vi "IR121206 Traitement Enr Npectre_SD.vi"(1 "Moyenne par pas":i8=4, 3 "resultat_input":dbl[](array[numeric])=array[24576 elements]) -> (0 "BgSig":dbl[][](array[numeric]), 2 "Ref-Bg":dbl[][](array[numeric]), 4 "BgRef":dbl[][](array[numeric]), 5 "Sig-Bg":dbl[][](array[numeric]))   [LabVIEW 2015]
panel:
  out "Graphe":dbl[](graph)
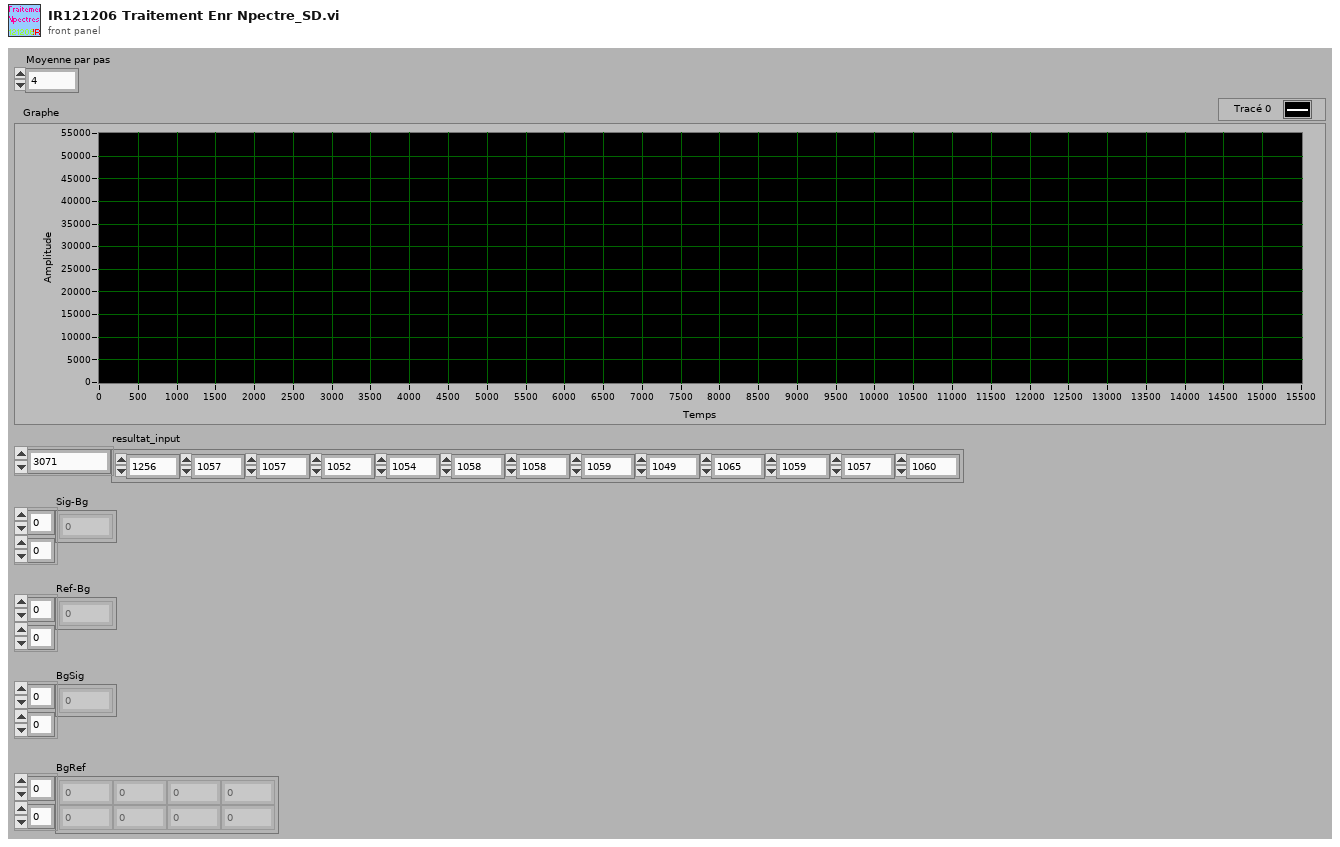
[diagram p1: front panel]
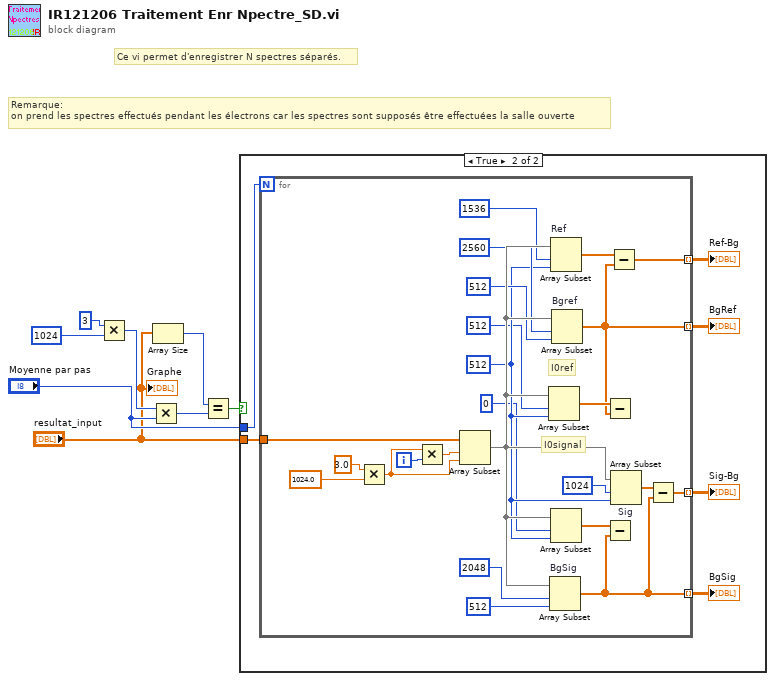
[diagram p0: block diagram]
diagram:
  # "Ce vi permet d'enregistrer N spectres séparés."
  # "Remarque: \non prend les spectres effectués pendant les électrons car les spectres sont supposés être effectuées la salle ouverte"
  n1 = Multiply(x=3, y=1024) -> (x*y=w6:i32)
  n2 = Multiply(x=w6, y="Moyenne par pas") -> (x*y=w4:i32)
  n3 = Array Size(array="resultat_input") -> (size(s)=w5:i32)
  n4 = Equal?(x=w5, y=w4) -> (x = y?=w3:bool)
  n5 = case shown="True" w3 {
    tunnel: "resultat_input" -> [_ w14]
    tunnel: "Moyenne par pas" -> [_ w13]
    frame False {
    }
    frame True {
      n6 = for {
        N: w13 -> [_]
        tunnel: w14 -> [w36]
        tunnel: [w18] -> w11 mode=indexing
        tunnel: [w17] -> w10 mode=indexing
        tunnel: [w16] -> w9 mode=indexing
        tunnel: [w15] -> w12 mode=indexing
        i -> [w24]
        w23 = 512 ("longueur")
        # "I0signal"
        # "I0ref"
        n7 = Multiply(x=3.0, y=1024.0) -> (x*y=w34:dbl)
        n8 = Multiply(x=w34, y=w24) -> (x*y=w35:dbl)
        n9 = Array Subset(array=w36, index=w35, length=w34) -> (w29:dbl[])
        n10 = Array Subset(array=w29, index=512 ("indice"), length=w23) -> (w30:dbl[])
        n11 = Array Subset "BgSig"(array=w29, index=2048 ("indice"), length=512 ("longueur")) -> (w16:dbl[])
        n12 = Array Subset "Ref"(array=w29, index=1536 ("indice"), length=w23) -> (w32:dbl[])
        n13 = Array Subset(array=w29, index=0 ("indice"), length=w23) -> (w31:dbl[])
        n14 = Array Subset "Bgref"(array=w29, index=2560 ("indice"), length=512 ("longueur")) -> (w15:dbl[])
        n15 = Subtract(x=w30, y=w15) -> ()  [unwired: 1 out]
        n16 = Subtract(x=w31, y=w16) -> ()  [unwired: 1 out]
        n17 = Subtract(x=w32, y=w15) -> (x-y=w17:dbl[])
        n18 = Array Subset "Sig"(array=w29, index=1024 ("indice"), length=w23) -> (w33:dbl[])
        n19 = Subtract(x=w33, y=w16) -> (x-y=w18:dbl[])
      }
      "Sig-Bg" <- w11
      "Ref-Bg" <- w10
      "BgSig" <- w9
      "BgRef" <- w12
    }
  }
  "Graphe" <- "resultat_input"
